vi "Do Core.vi"(8 "error in (no error)":errorcluster, 9 "Actor in":refnum<class "Actor.lvclass">, 11 "Reply Message":refnum<class "Get Table Msg.lvclass">) -> (0 "error out":errorcluster, 1 "Actor out":refnum<class "Actor.lvclass">, 2 "Reply":variant)   [LabVIEW 2020, in "Panel Form Controller.lvlib" / "Get Table Msg.lvclass"]
doc: "(<B>Filename</B>: Actor Framework.lvlib:Reply Msg.lvclass:Do Core.vi)\n\nDefines what an actor does when it receives <B>Reply Message</B>. This method also defines the <B>Reply</B> that is returned to the actor that sent <B>Reply Message</B>.\n\nBy default, this method does nothing, and <B>Reply</B> is the ancestor Message class. A child class must override this method to define behavior and specify a child of the Message class to return in the <B>Reply</B> output."
uses:
  Get Table Msg.lvclass
  <vilib>/ActorFramework/Actor/Actor.lvclass
  Form Controller/Panel Form Controller.lvclass
  C:/Program Files (x86)/National Instruments/LabVIEW 2020/vi.lib/ActorFramework/Actor/Actor.lvclass
  77e6804e-9d25-4444-9c60-0f0c9d8c69c1.vi
  Database OOP/Table Libraries/Basic Table/Basic Table Class/Basic Table.lvclass
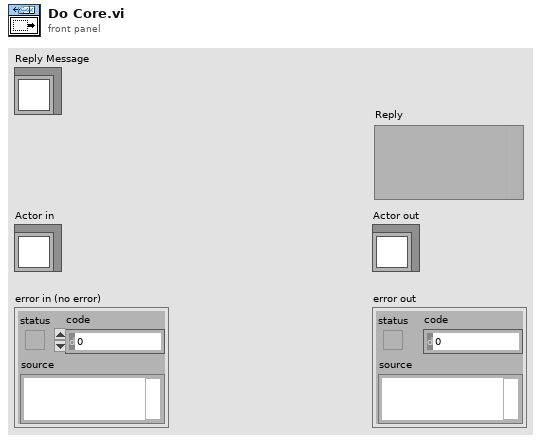
[diagram p1: front panel]
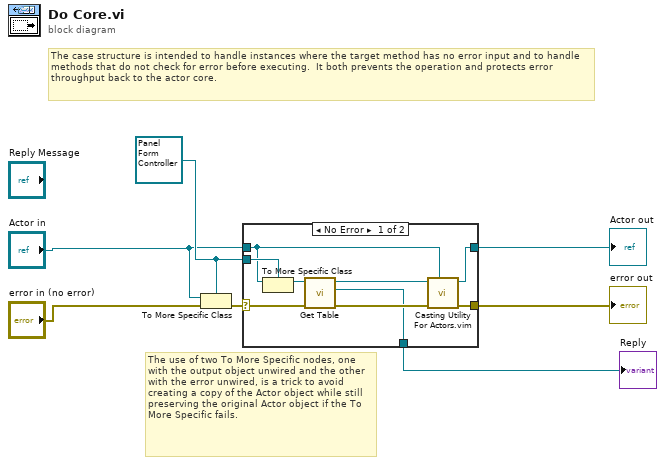
[diagram p0: block diagram]
diagram:
  w6 = refnum<class "Panel Form Controller.lvclass"> refnum ("Actor in")
  # "The use of two To More Specific nodes, one with the output object unwired and the other with the error unwired, is a trick to avoid creating a copy of the Actor object while still preserving the original Actor object if the To More Specific fails."
  # "The case structure is intended to handle instances where the target method has no error input and to handle methods that do not check for error before executing.  It both prevents the operation and protects error throughput back to the actor core."
  n1 = To More Specific Class(target class=w6, reference="Actor in", error in="error in (no error)") -> (error out=w7:errorcluster)  [unwired: 1 out]
  n2 = case shown="No Error" w7 {
    selector: w7 -> [w16 w18]
    tunnel: [w10 w18] -> w3
    tunnel: [w11 w17] -> w2
    tunnel: "Actor in" -> [w13 w17]
    tunnel: w6 -> [w14 _]
    tunnel: [w8 _] -> w1
    frame No Error {
      n3 = To More Specific Class(target class=w14, reference=w13) -> (specific class reference=w15:refnum<class "Panel Form Controller.lvclass">)  [unwired: 1 in, 1 out]
      n4 = call-dynamic "Get Table.vi"("error in (no error)"=w16, "Panel Form Controller in"=w15) -> ("error out"=w9:errorcluster, "Table"=w8:refnum<class "Basic Table.lvclass">, "Panel Form Controller out"=w12:refnum<class "Panel Form Controller.lvclass">)  [unwired: 7 in]
      n5 = call "Casting Utility For Actors.vim"("type"=w13, "error in (no error)"=w9, "Actor in"=w12) -> ("error out"=w10:errorcluster, "Actor out"=w11:refnum<class "Actor.lvclass">)  [unwired: 7 in]
    }
    frame Error {
      # "If type check fails, pass the original object out again."
    }
  }
  "error out" <- w3
  "Actor out" <- w2
  "Reply" <- w1
